vi "SetVelocity.vi"() -> ()   [LabVIEW 2011]
uses:
  Robot Global Data.vi
  <vilib>/addons/control/pid/pid.llb/PID (DBL).vi
  <vilib>/addons/control/pid/NI_PID_pid.lvlib
panel:
  out "Zero?":dbl
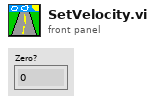
[diagram p1: front panel]
types:
  T1 = typedef "WPI_MotorControlDeviceRef.ctl" = cluster{"DeviceStatus":errorcluster, "Type":enum16{"PWM", "CAN"}, "PWM":cluster{"Digital Module":T2, "PWM Channel":T3, "DeadBand":T4}, "CAN":cluster{"Device Number":u8, "Control Mode":T5, "Semaphore":T6, "Max Vout":dbl}, "Invert":bool, "TransformRef":T7, "InvTransformRef":T7}
  T2 = typedef "FPGA_TypedefDigitalModule.ctl" = enum16{"Digital Module 1", "Digital Module 2"}
  T3 = typedef "FPGA_DIOPWMChannel.ctl" = enum8{"PWM 1", "PWM 2", "PWM 3", "PWM 4", "PWM 5", "PWM 6", "PWM 7", "PWM 8", "PWM 9", "PWM 10", "Invalid"}
  T4 = typedef "WPI_PWMDeadband.ctl" = cluster{"Name":string, "maxPositivePwm":i32, "minPositivePwm":i32, "centerPwm":i32, "maxNegativePwm":i32, "minNegativePwm":i32, "angularRange":u16}
  T5 = typedef "WPI_CANJaguar_ControlMode.ctl" = enum8{"Percent VBus", "Current", "Speed", "Position", "Voltage"}
  T6 = typedef "Semaphore RefNum" = refnum<k1>
  T7 = typedef "WPI_PWMTransform_ConPane.ctl" = refnum<vi>
  T8 = cluster{"proportional gain (Kc)":dbl, "integral time (Ti, min)":dbl, "derivative time (Td, min)":dbl}
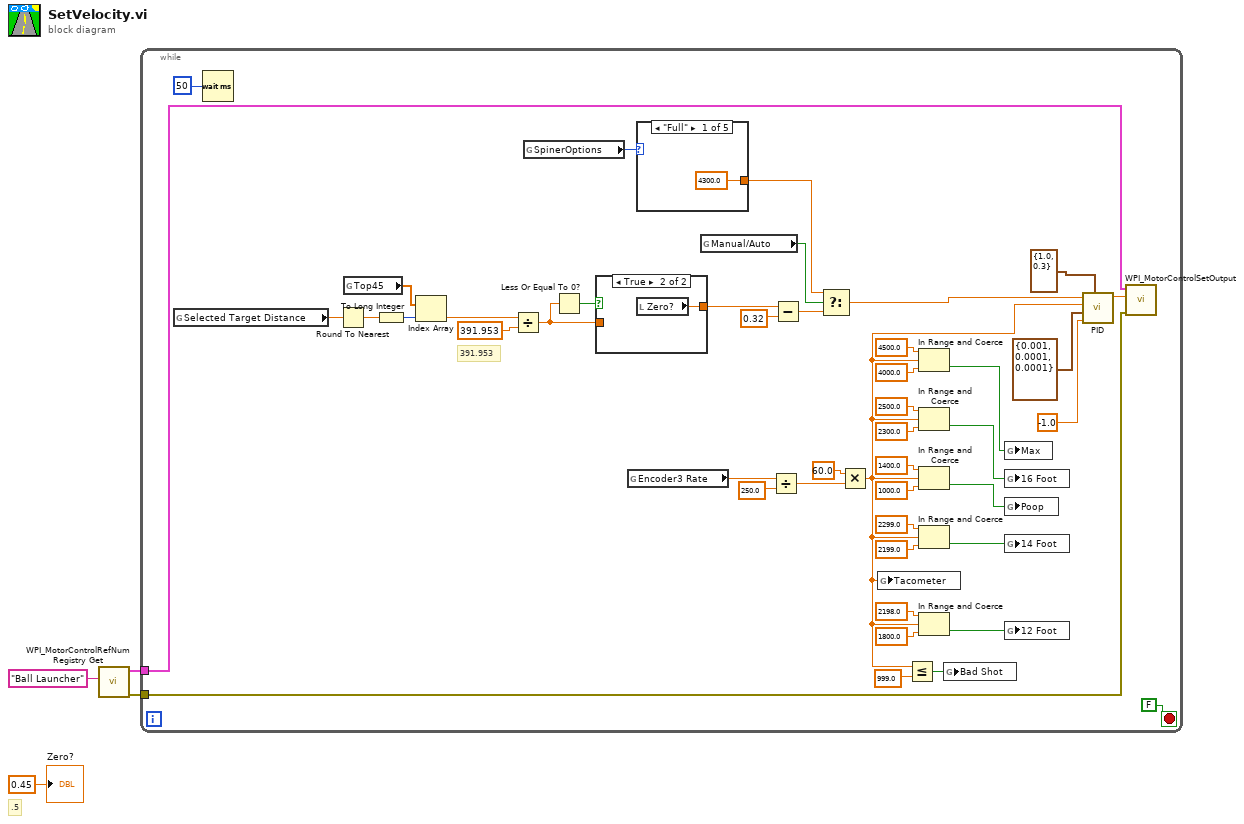
[diagram p0: block diagram]
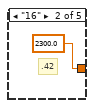
[diagram p2: hidden frame]
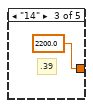
[diagram p3: hidden frame]
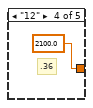
[diagram p4: hidden frame]
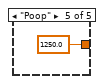
[diagram p5: hidden frame]
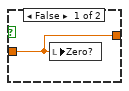
[diagram p6: hidden frame]
diagram:
  # ".5"
  n1 = call <vilib>:"WPI_MotorControlRefNum Registry Get.vi"("refnum name"="Ball Launcher") -> ("error out"=w2:errorcluster, "MotorControlDevRef"=w3:T1)  [unwired: 9 in]
  n2 = while {
    tunnel: w3 -> [w49]
    tunnel: w2 -> [w48]
    stop <- FALSE stop-if-true
    # "391.953"
    n3 = global read "Robot Global Data.vi" "Selected Target Distance"() -> (w37:dbl)
    n4 = Wait (ms)(milliseconds to wait=50) -> ()  [unwired: 1 out]
    n5 = Round To Nearest(number=w37) -> (nearest integer value=w36:dbl)
    n6 = global read "Robot Global Data.vi" "Top45"() -> (w38:dbl[])
    n7 = To Long Integer(number=w36) -> (32bit integer=w35:i32)
    n8 = Index Array(array=w38, index=w35) -> (element=w33:dbl)
    n9 = Divide(x=w33, y=391.953) -> (x/y=w44:dbl)
    n10 = global read "Robot Global Data.vi" "SpinerOptions"() -> (w41:enum16{"Full", "16", "14", "12", "Poop"})
    n11 = Less Or Equal To 0?(x=w44) -> (x <= 0?=w45:bool)
    n12 = case shown="True" w45 {
      tunnel: w44 -> [w55 _]
      tunnel: [w55 w56] -> w31
      frame False {
        n13 = local write "Zero?"(w55) -> ()
      }
      frame True {
        n14 = local read "Zero?"() -> (w56:dbl)
      }
    }
    n15 = global read "Robot Global Data.vi" "Encoder3 Rate"() -> (w28:dbl)
    n16 = case shown="\"Full\"" w41 {
      tunnel: [4300.0 2300.0 2200.0 2100.0 1250.0] -> w39
      frame "Full" {
      }
      frame "16" {
        # ".42"
      }
      frame "14" {
        # ".39"
      }
      frame "12" {
        # ".36"
      }
      frame "Poop" {
      }
    }
    n17 = global read "Robot Global Data.vi" "Manual/Auto"() -> (w32:bool)
    n18 = Divide(x=w28, y=250.0) -> (x/y=w26:dbl)
    n19 = Subtract(x=w31, y=0.32) -> (x-y=w29:dbl)
    n20 = Select(t=w39, s=w32, f=w29) -> (s? t:f=w6:dbl)
    n21 = Multiply(x=60.0, y=w26) -> (x*y=w5:dbl)
    n22 = global write "Robot Global Data.vi" "Tacometer"(w5) -> ()
    n23 = Less Or Equal?(x=w5, y=999.0) -> (x <= y?=w7:bool)
    n24 = In Range and Coerce(upper limit=4500.0, x=w5, lower limit=4000.0) -> (In Range?=w8:bool)  [unwired: 1 out]
    n25 = In Range and Coerce(upper limit=2500.0, x=w5, lower limit=2300.0) -> (In Range?=w9:bool)  [unwired: 1 out]
    n26 = In Range and Coerce(upper limit=1400.0, x=w5, lower limit=1000.0) -> (In Range?=w12:bool)  [unwired: 1 out]
    n27 = In Range and Coerce(upper limit=2299.0, x=w5, lower limit=2199.0) -> (In Range?=w10:bool)  [unwired: 1 out]
    n28 = In Range and Coerce(upper limit=2198.0, x=w5, lower limit=1800.0) -> (In Range?=w11:bool)  [unwired: 1 out]
    n29 = global write "Robot Global Data.vi" "Bad Shot"(w7) -> ()
    n30 = global write "Robot Global Data.vi" "Max"(w8) -> ()
    n31 = global write "Robot Global Data.vi" "16 Foot"(w9) -> ()
    n32 = global write "Robot Global Data.vi" "Poop"(w12) -> ()
    n33 = global write "Robot Global Data.vi" "14 Foot"(w10) -> ()
    n34 = global write "Robot Global Data.vi" "12 Foot"(w11) -> ()
    n35 = call-poly <vilib>:"PID.vi"("output range"=cluster{"output high":dbl, "output low":dbl} {"output high"=1.0, "output low"=0.3}, "dt (s)"=-1.0, "PID gains"=T8 {"proportional gain (Kc)"=0.001, "integral time (Ti, min)"=0.0001, "derivative time (Td, min)"=0.0001}, "process variable"=w5, "setpoint"=w6) -> ("output"=w24:dbl)  [unwired: 5 in, 1 out]
    n36 = call <vilib>:"WPI_MotorControlSetOutput.vi"("error in (no error)"=w48, "Output"=w24, "MotorControlDevRef"=w49) -> ()  [unwired: 7 in, 2 out]
  }
  "Zero?" <- 0.45 ("Zero?")
